vi "AI Array Add or Remove.vi"(8 "error in (no error)":errorcluster, 10 "Size":i32, 11 "Configuration.Channels.AI":T1 {"References" items=["", "1", "2", "3"]; "Channel" min=1}) -> (0 "error out":errorcluster, 3 "Configuration.Channels.AI":T1 {"References" items=["", "1", "2", "3"]; "Channel" min=1})   [LabVIEW 2019, in "Instrument.DAQ.lvclass"]
uses:
  Instrument.DAQ.lvclass
  Typedefs/AI.Channel--Cluster--Array.ctl
  Typedefs/AI.Channel--Cluster.ctl
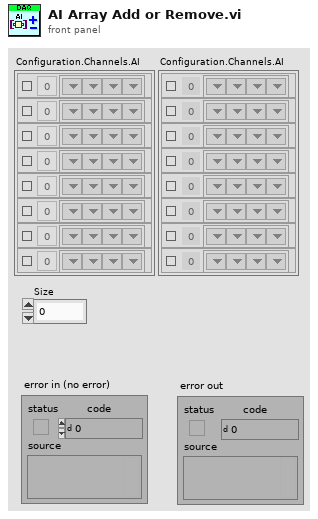
[diagram p1: front panel]
types:
  T1 = typedef "Instrument.DAQ.lvclass/AI.Channel--Cluster--Array.ctl" = T2[]
  T2 = typedef "Instrument.DAQ.lvclass/AI.Channel--Cluster.ctl" = cluster{"Enable?":bool, "Channel":i32, "References":i32[]}
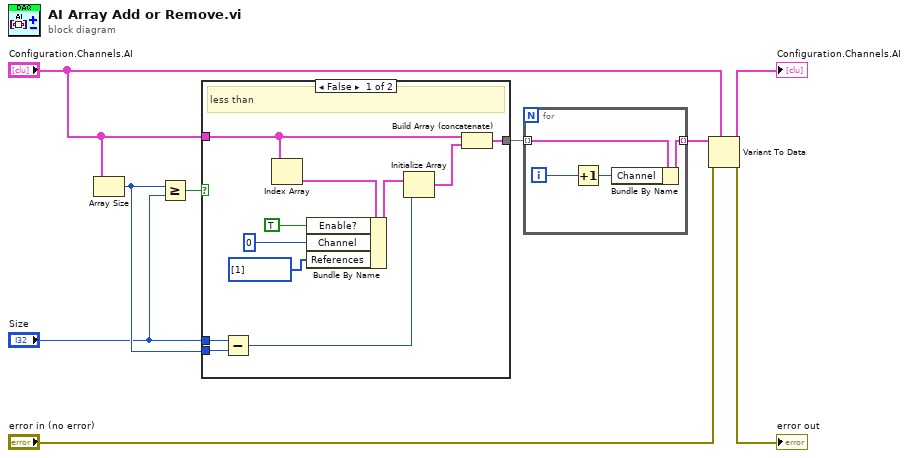
[diagram p0: block diagram]
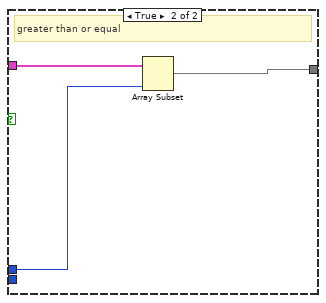
[diagram p2: hidden frame]
diagram:
  n1 = Array Size(array="Configuration.Channels.AI") -> (size(s)=w9:i32)
  n2 = Greater Or Equal?(x=w9, y="Size") -> (x >= y?=w8:bool)
  n3 = case shown="False" w8 {
    tunnel: "Configuration.Channels.AI" -> [w11 w23]
    tunnel: "Size" -> [w18 w22]
    tunnel: [w19 w21] -> w6
    tunnel: w9 -> [w17 _]
    frame False {
      # "less than"
      n4 = Subtract(x=w18, y=w17) -> (x-y=w16:i32)
      n5 = Index Array(array=w11) -> (element=w10:T2)  [unwired: 1 in]
      n6 = Bundle By Name(cluster=w10, "Enable?"=TRUE, "Channel"=0, "References"=i32[] [1]) -> (w15:T2)
      n7 = Initialize Array(w15, w16) -> (w20:T2[])
      n8 = Build Array (concatenate)(w11, w20) -> (w19:T1)
    }
    frame True {
      # "greater than or equal"
      n9 = Array Subset(array=w23, length=w22) -> (w21:T1)  [unwired: 1 in]
    }
  }
  n10 = for {
    tunnel: w6 -> [w27] mode=indexing
    tunnel: [w26] -> w5 mode=indexing
    i -> [w24]
    n11 = Increment(x=w24) -> (x+1=w25:i32)
    n12 = Bundle By Name(cluster=w27, "Channel"=w25) -> (w26:T2)
  }
  n13 = Variant To Data(error in="error in (no error)", type="Configuration.Channels.AI", Variant=w5) -> (data=→"Configuration.Channels.AI":T1, error out=→"error out":errorcluster)
